vi "close.vi"(8 "error in (no error)":errorcluster, 11 "k3390_AWG in":refnum<class "k3390_AWG.lvclass">) -> (0 "error out":errorcluster)   [LabVIEW 2009, in "Hardware.lvlib" / "Channels.lvlib" / "k3390_AWG.lvclass"]
uses:
  k3390_AWG.lvclass
  k3390_AWG.lvclass/k3390_AWG.ctl
  <instrlib>/Keithley 3390/Keithley 3390.lvlib
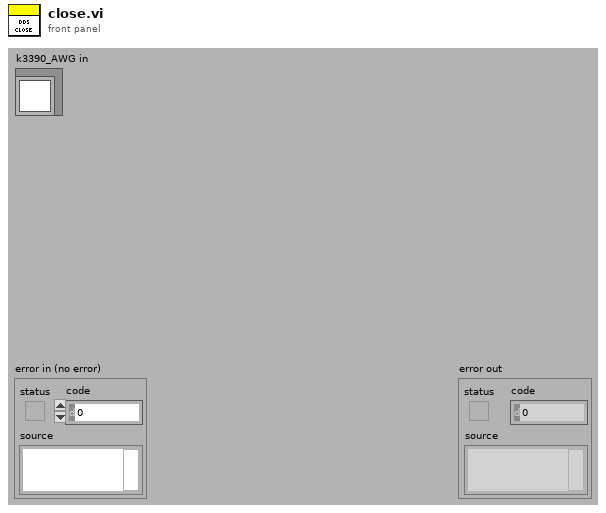
[diagram p1: front panel]
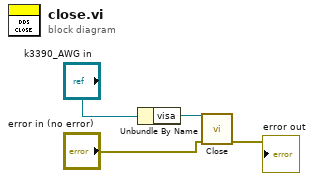
[diagram p0: block diagram]
diagram:
  n1 = Unbundle By Name("k3390_AWG in") -> ("visa"=w1:refnum<visa-resource-name>)
  n2 = call <instrlib>:"Close.vi"("error in (no error)"="error in (no error)", "VISA resource name"=w1) -> ("error out"=→"error out":errorcluster)  [unwired: 9 in]
